vi "Call.vi"(7 "Actor in":refnum<class "Actor.lvclass">, 8 "Error in":errorcluster, 9 "Parent Stopped":bool, 10 "Safe Stop":bool=TRUE) -> (0 "Error out":errorcluster, 5 "Actor out":refnum<class "Actor.lvclass">)   [LabVIEW 2025, in "jettl.lvlib" / "Stop Msg.lvlib"]
uses:
  Stop Msg.lvlib
  Actor/Actor.lvclass
  Stop Msg/Stop Msg.lvclass
  C:/git/jettl/src/jettl/jettl/Msg/Msg.lvclass
  jettl.lvlib
  Stop Msg Output/Stop Msg Output.lvclass
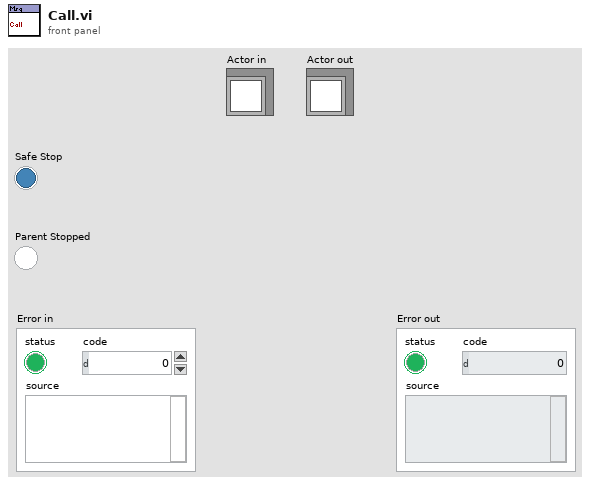
[diagram p1: front panel]
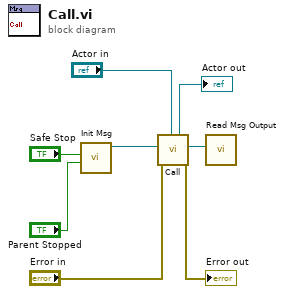
[diagram p0: block diagram]
diagram:
  n1 = call "Init Msg.vi"("Parent Stopped"="Parent Stopped", "Safe Stop"="Safe Stop") -> ("Stop Msg out"=w7:refnum<class "Stop Msg.lvclass">)  [unwired: 9 in]
  n2 = call "Call.vi"("Actor in"="Actor in", "Error in"="Error in", "Msg"=w7) -> ("Error out"=→"Error out":errorcluster, "Msg Output"=w3:refnum<class "Msg Output.lvclass">, "Actor out"=→"Actor out":refnum<class "Actor.lvclass">)  [unwired: 6 in]
  n3 = call "Read Msg Output.vi"("Msg Output"=w3) -> ()  [unwired: 11 in]
